vi "MGCC_StaEst_initial_5.vi"() -> ()   [LabVIEW 2016]
panel:
  out "StateVar":dbl[](array[numeric])
  out "InitialValue":dbl[](array[numeric])
  out "Weight":dbl[][](array[numeric])
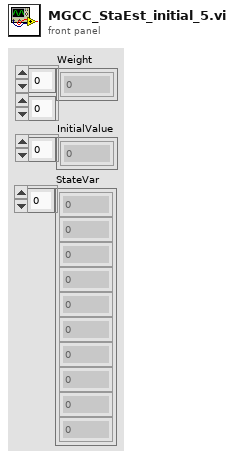
[diagram p1: front panel]
types:
  T1 = cluster{"Node":dbl, "Line":dbl, "StateVar":i32, "Zeroinj":i32}
  T2 = cluster{"VOL":cdb[][], "PN":dbl[][], "QN":dbl[][], "IN":dbl[][], "Ve":dbl[][], "Vf":dbl[][], "VN":dbl[][], "AN":dbl[][]}
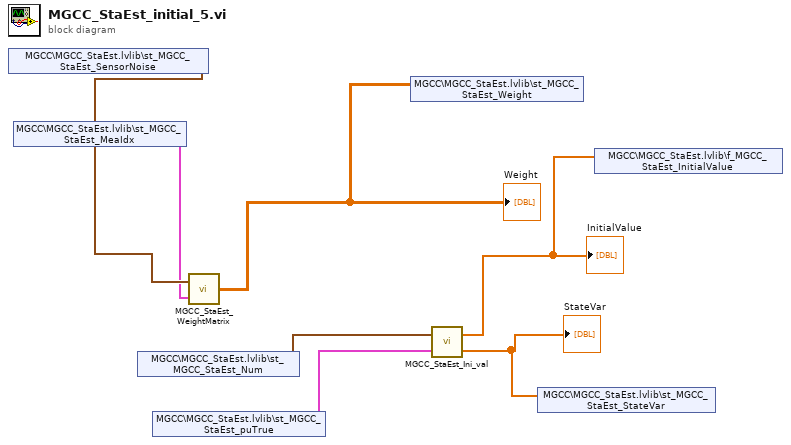
[diagram p0: block diagram]
diagram:
  n1 = shared-variable "MGCC\\MGCC_StaEst.lvlib\\st_MGCC_StaEst_SensorNoise"() -> (w5:cluster{"PN":dbl, "QN":dbl, "VN":dbl})  [unwired: 1 in, 1 out]
  n2 = shared-variable "MGCC\\MGCC_StaEst.lvlib\\st_MGCC_StaEst_MeaIdx"() -> (w4:cluster{"PN":dbl[], "QN":dbl[], "VN":dbl[]})  [unwired: 1 in, 1 out]
  n3 = shared-variable "MGCC\\MGCC_StaEst.lvlib\\st_MGCC_StaEst_Num"() -> (w7:T1)  [unwired: 1 in, 1 out]
  n4 = shared-variable "MGCC\\MGCC_StaEst.lvlib\\st_MGCC_StaEst_puTrue"() -> (w6:T2)  [unwired: 1 in, 1 out]
  n5 = call "MGCC_StaEst_WeightMatrix.vi"("MeaIdx"=w4, "SensorError"=w5) -> ("R"=w3:dbl[][])
  "Weight" <- w3
  n6 = shared-variable "MGCC\\MGCC_StaEst.lvlib\\st_MGCC_StaEst_Weight"(w3) -> ()  [unwired: 1 in, 1 out]
  n7 = call "MGCC_StaEst_Ini_val.vi"("puTrue"=w6, "Num"=w7) -> ("StateVar_true"=w1:dbl[], "InitialValue"=w2:dbl[])
  "InitialValue" <- w2
  "StateVar" <- w1
  n8 = shared-variable "MGCC\\MGCC_StaEst.lvlib\\st_MGCC_StaEst_StateVar"(w1) -> ()  [unwired: 1 in, 1 out]
  n9 = shared-variable "MGCC\\MGCC_StaEst.lvlib\\f_MGCC_StaEst_InitialValue"(w2) -> ()  [unwired: 1 in, 1 out]
